vi "Op-Upload Trace.vi"(8 "error in (no error)":errorcluster, 9 "trace":dbl[](array[numeric]) format="%^.3e", 10 "trace (variable) name":string, 11 "VISA session":refnum<visa-resource-name>) -> (0 "error out":errorcluster, 3 "VISA resource name out":refnum<visa-resource-name>)   [LabVIEW 2016, in "Agilent 415X Series.lvlib"]
doc: "This VI loads a trace into one of the user defined variables.\n\nNo error checking is peformed by this VI since the instrument will catch all the data problems and report them into the error queue. To read the instrument's error queue, run \"HP415xA Sys-Error Query.vi\"."
uses:
  Agilent 415X Series.lvlib
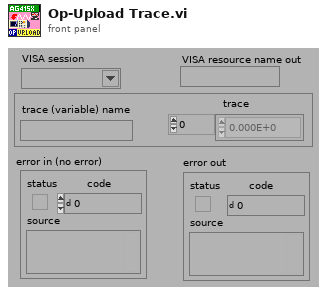
[diagram p1: front panel]
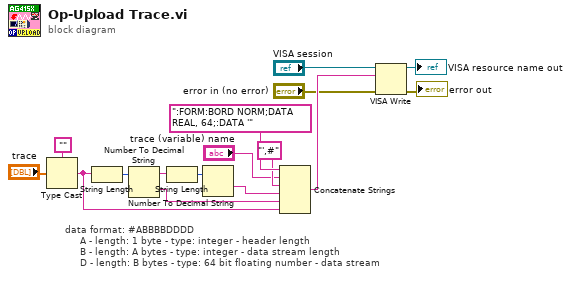
[diagram p0: block diagram]
diagram:
  # "data format: #ABBBBDDDD \n     A - length: 1 byte - type: integer - header length\n     B - length: A bytes - type: integer - data stream length\n     D - length: B bytes - type: 64 bit floating number - data stream"
  n1 = Type Cast(type="", x="trace") -> (*(type *) &x=w3:string)
  n2 = String Length(string=w3) -> (length=w7:i32)
  n3 = Number To Decimal String(number=w7) -> (decimal integer string=w5:string)  [unwired: 1 in]
  n4 = String Length(string=w5) -> (length=w6:i32)
  n5 = Number To Decimal String(number=w6) -> (decimal integer string=w4:string)  [unwired: 1 in]
  n6 = Concatenate Strings(":FORM:BORD NORM;DATA REAL, 64;:DATA '", "trace (variable) name", "',#", w4, w5, w3) -> (w14:string)
  n7 = VISA Write(VISA resource name="VISA session", write buffer=w14, error in (no error)="error in (no error)") -> (VISA resource name out=→"VISA resource name out":refnum<visa-resource-name>, error out=→"error out":errorcluster)  [unwired: 1 out]
